vi "AI Configure Channel.vi"(5 "Samples per channel":sgl=1.0, 8 "error in (no error)":errorcluster, 10 "Sampe Rate":sgl=1000.0, 11 "MicroDAQ.lvlib:Analog Input.lvclass":refnum<class "Analog Input.lvclass">) -> (0 "error out":errorcluster, 3 "MicroDAQ.lvlib:Analog Input.lvclass out":refnum<class "Analog Input.lvclass">)   [LabVIEW 2009, in "MicroDAQ.lvlib" / "Analog Input.lvclass"]
doc: "Sets the rate of the Sample Clock, and the number of samples to acquire (use -1 for continous acquisition). If you choose blocking opiton, Read.VI will block execution until all samples are acquired. In non-blocking mode Read.VI will read buffor immediatly, no mater how many samples were acquired."
uses:
  <instrlib>/MicroDAQ/Channel/Analog Input/Analog Input.lvclass
  <instrlib>/MicroDAQ/Channel/Analog Input/Analog Input.lvclass/Analog Input.ctl
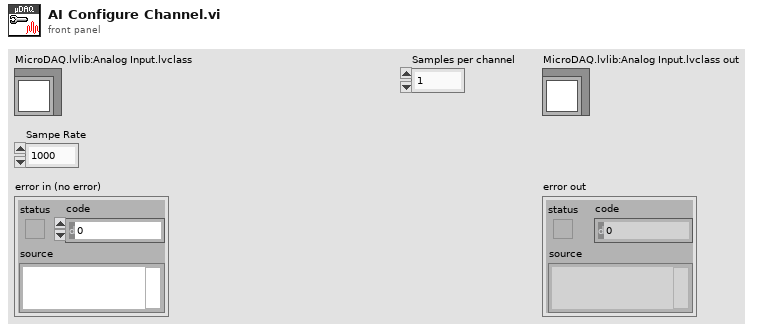
[diagram p1: front panel]
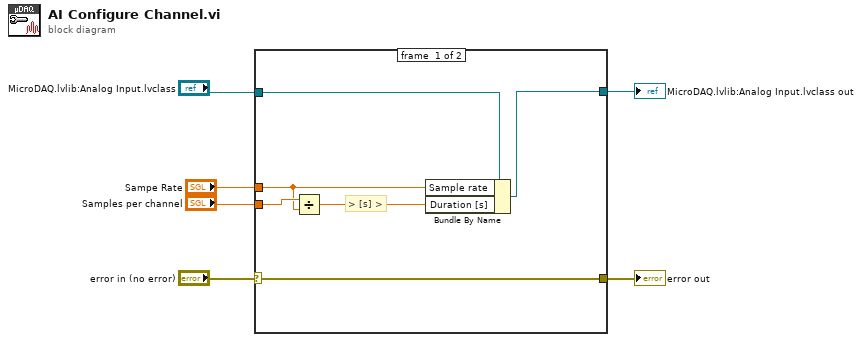
[diagram p0: block diagram]
diagram:
  n1 = case shown="No Error" "error in (no error)" {
    selector: "error in (no error)" -> [w10 w13]
    tunnel: [w10 w13] -> w5
    tunnel: [w11 w14] -> w4
    tunnel: "MicroDAQ.lvlib:Analog Input.lvclass" -> [w12 w14]
    tunnel: "Sampe Rate" -> [w8 _]
    tunnel: "Samples per channel" -> [w9 _]
    frame #0 {
      # "> [s] >"
      n2 = Divide(x=w9, y=w8) -> (x/y=w7:sgl)
      n3 = Bundle By Name(cluster=w12, "Sample rate"=w8, "Duration [s]"=w7) -> (w11:refnum<class "Analog Input.lvclass">)
    }
    frame #1 {
    }
  }
  "error out" <- w5
  "MicroDAQ.lvlib:Analog Input.lvclass out" <- w4
